vi "ENPH354_A2Q4_20213140.vi"() -> ()   [LabVIEW 2020]
panel:
  out "d":bool
  out "e":bool
  out "f":bool
  out "g":bool
  out "c":bool
  out "b":bool
  out "a":bool
  in  "stop":bool
  # "Author: Jose Ramon Gonzalez\nENPH354 Assignment 2 Q4"
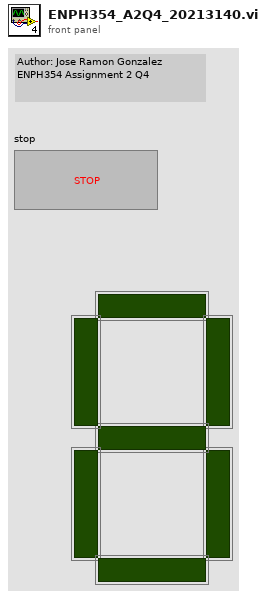
[diagram p1: front panel]
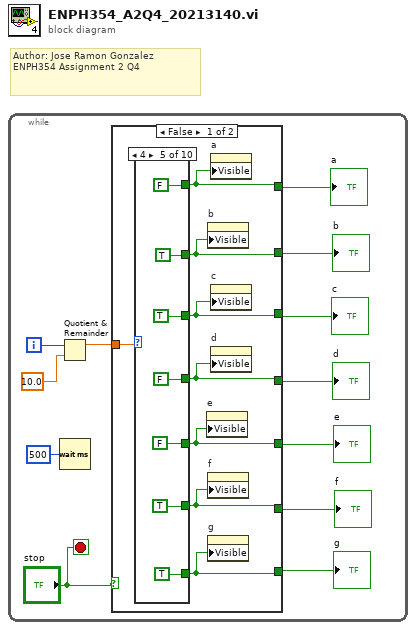
[diagram p0: block diagram]
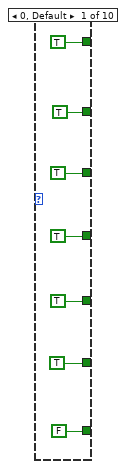
[diagram p2: hidden frame]
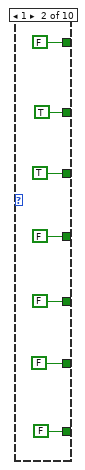
[diagram p3: hidden frame]
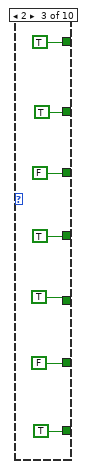
[diagram p4: hidden frame]
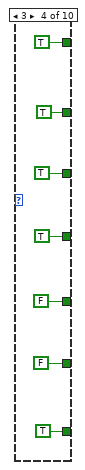
[diagram p5: hidden frame]
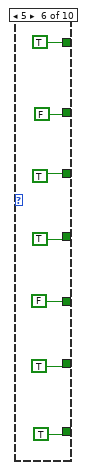
[diagram p6: hidden frame]
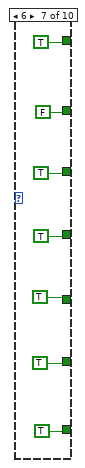
[diagram p7: hidden frame]
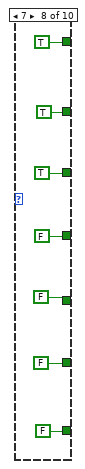
[diagram p8: hidden frame]
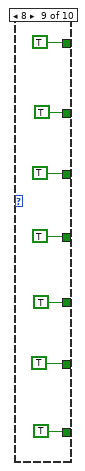
[diagram p9: hidden frame]
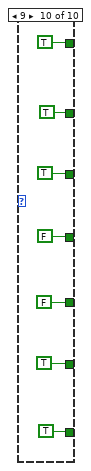
[diagram p10: hidden frame]
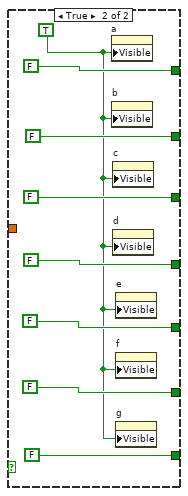
[diagram p11: hidden frame]
diagram:
  # "Author: Jose Ramon Gonzalez\nENPH354 Assignment 2 Q4"
  n1 = while {
    i -> [w9]
    stop <- "stop" stop-if-true
    n2 = Quotient & Remainder(x=w9, y=10.0) -> (x-y*floor(x/y)=w11:dbl)  [unwired: 1 out]
    n3 = Wait (ms)(milliseconds to wait=u32 500) -> ()  [unwired: 1 out]
    n4 = case shown="False" "stop" {
      tunnel: [w15 FALSE] -> w7
      tunnel: [w13 FALSE] -> w6
      tunnel: [w14 FALSE] -> w5
      tunnel: [w16 FALSE] -> w4
      tunnel: [w17 FALSE] -> w3
      tunnel: [w18 FALSE] -> w2
      tunnel: [w19 FALSE] -> w1
      tunnel: w11 -> [w20 _]
      frame False {
        n5 = case shown="4" w20 {
          tunnel: [TRUE FALSE TRUE TRUE FALSE TRUE TRUE TRUE TRUE TRUE] -> w15
          tunnel: [TRUE TRUE TRUE TRUE TRUE FALSE FALSE TRUE TRUE TRUE] -> w13
          tunnel: [TRUE TRUE FALSE TRUE TRUE TRUE TRUE TRUE TRUE TRUE] -> w14
          tunnel: [TRUE FALSE TRUE TRUE FALSE TRUE TRUE FALSE TRUE FALSE] -> w16
          tunnel: [TRUE FALSE TRUE FALSE FALSE FALSE TRUE FALSE TRUE FALSE] -> w17
          tunnel: [TRUE FALSE FALSE FALSE TRUE TRUE TRUE FALSE TRUE TRUE] -> w18
          tunnel: [FALSE FALSE TRUE TRUE TRUE TRUE TRUE FALSE TRUE TRUE] -> w19
          frame 0, Default {
          }
          frame 1 {
          }
          frame 2 {
          }
          frame 3 {
          }
          frame 4 {
          }
          frame 5 {
          }
          frame 6 {
          }
          frame 7 {
          }
          frame 8 {
          }
          frame 9 {
          }
        }
        n6 = property on="e" class="Bool (strict)"("Visible"=w17) -> ()  [unwired: 2 in, 2 out]
        n7 = property on="b" class="Bool (strict)"("Visible"=w13) -> ()  [unwired: 2 in, 2 out]
        n8 = property on="f" class="Bool (strict)"("Visible"=w18) -> ()  [unwired: 2 in, 2 out]
        n9 = property on="g" class="Bool (strict)"("Visible"=w19) -> ()  [unwired: 2 in, 2 out]
        n10 = property on="a" class="Bool (strict)"("Visible"=w15) -> ()  [unwired: 2 in, 2 out]
        n11 = property on="c" class="Bool (strict)"("Visible"=w14) -> ()  [unwired: 2 in, 2 out]
        n12 = property on="d" class="Bool (strict)"("Visible"=w16) -> ()  [unwired: 2 in, 2 out]
      }
      frame True {
        w91 = TRUE
        n13 = property on="a" class="Bool (strict)"("Visible"=w91) -> ()  [unwired: 2 in, 2 out]
        n14 = property on="b" class="Bool (strict)"("Visible"=w91) -> ()  [unwired: 2 in, 2 out]
        n15 = property on="c" class="Bool (strict)"("Visible"=w91) -> ()  [unwired: 2 in, 2 out]
        n16 = property on="d" class="Bool (strict)"("Visible"=w91) -> ()  [unwired: 2 in, 2 out]
        n17 = property on="e" class="Bool (strict)"("Visible"=w91) -> ()  [unwired: 2 in, 2 out]
        n18 = property on="f" class="Bool (strict)"("Visible"=w91) -> ()  [unwired: 2 in, 2 out]
        n19 = property on="g" class="Bool (strict)"("Visible"=w91) -> ()  [unwired: 2 in, 2 out]
      }
    }
    "a" <- w7
    "b" <- w6
    "c" <- w5
    "d" <- w4
    "e" <- w3
    "f" <- w2
    "g" <- w1
  }
